vi "UI.Connection.State.Get.vi"(6 "Menu Ref":refnum<k9>, 7 "Name Ref":refnum<vi>, 8 "error in (no error)":errorcluster, 9 "Addon Path in":string, 10 "NIVS.System Definition Root in":refnum<k24>, 11 "NIVS.Workspace Ref in":T1) -> (0 "error out":errorcluster, 1 "Addon Connected?":bool, 2 "NIVS.System Definition Root out":refnum<k24>, 3 "NIVS.Workspace Ref out":T1)   [LabVIEW 2019, in "J1939 Workspace Shared.lvlib"]
uses:
  J1939 Workspace Shared.lvlib
  <vilib>/NI VeriStand/Execution/Workspace/WorkspaceAPI.ctl
  NationalInstruments.VeriStand.ClientAPI
  NationalInstruments.VeriStand.SystemStorage
  NationalInstruments.VeriStand.SystemDefinitionAPI
  <vilib>/NI VeriStand/Execution/Workspace/NI_VS Workspace ExecutionAPI.lvlib
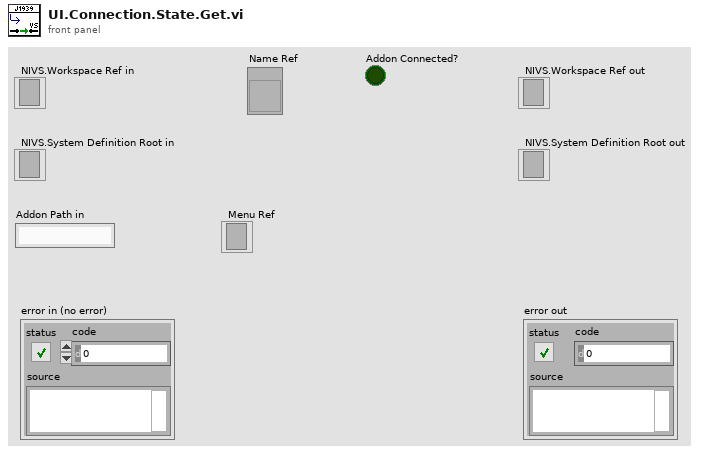
[diagram p1: front panel]
types:
  T1 = typedef "NI_VS Workspace ExecutionAPI.lvlib/WorkspaceAPI.ctl" = refnum<k24>
  T2 = typedef "NI_VS Workspace ExecutionAPI.lvlib/SystemState.ctl" = u8
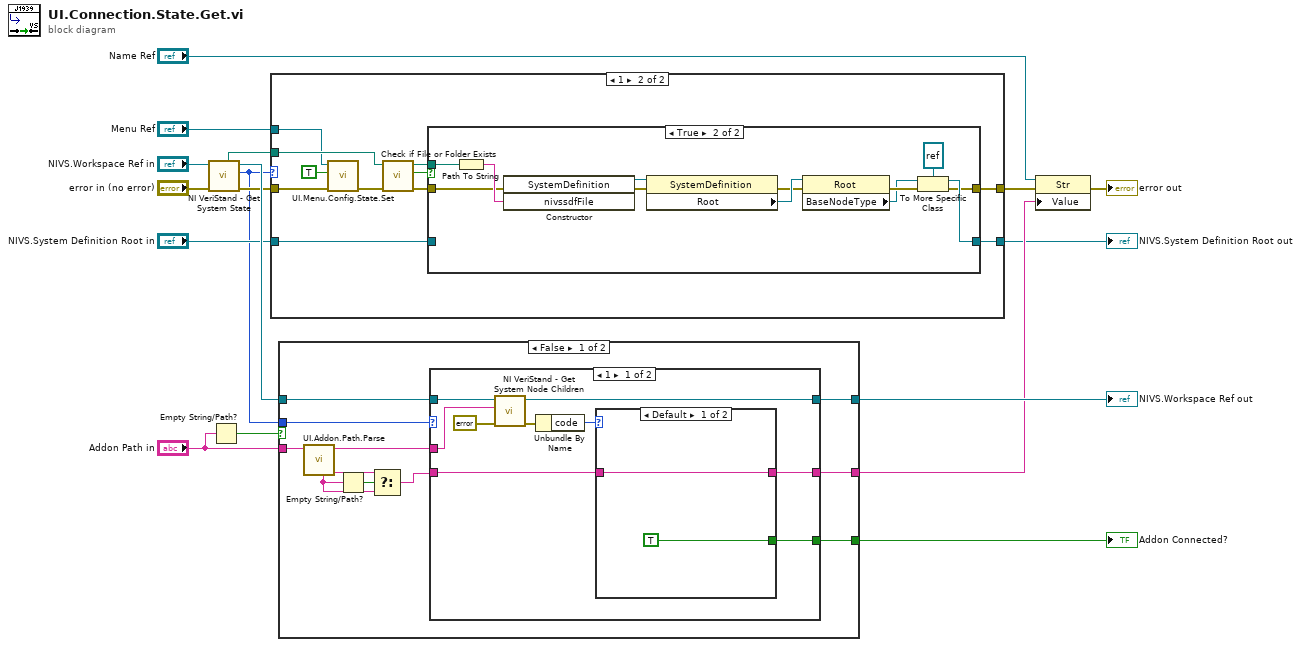
[diagram p0: block diagram]
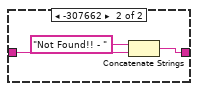
[diagram p2: hidden frame]
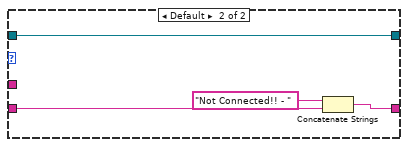
[diagram p3: hidden frame]
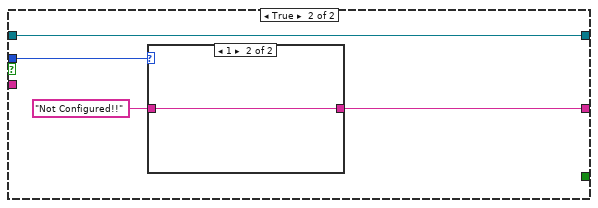
[diagram p4: hidden frame]
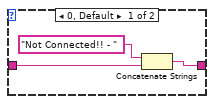
[diagram p5: hidden frame]
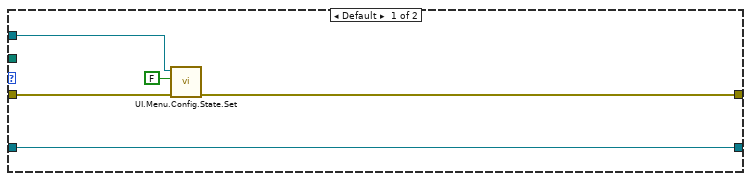
[diagram p6: hidden frame]
diagram:
  n1 = call <vilib>:"NI VeriStand - Get System State.vi"("error in (no error)"="error in (no error)", "WorkspaceManager in"="NIVS.Workspace Ref in") -> ("error out"=w5:errorcluster, "System State"=w2:T2, "WorkspaceManager  out"=w8:T1, "System Definition File"=w4:path)  [unwired: 5 in, 1 out]
  n2 = Empty String/Path?(string/path="Addon Path in") -> (empty?=w14:bool)
  n3 = case shown="1" w2 {
    tunnel: [w22 w33] -> w7
    tunnel: [w20 w32] -> w3
    tunnel: "NIVS.System Definition Root in" -> [w22 w29]
    tunnel: w5 -> [w19 w24]
    tunnel: w4 -> [_ w28]
    tunnel: "Menu Ref" -> [w18 w23]
    frame Default {
      n4 = call "UI.Menu.Config.State.Set.vi"("error in (no error)"=w19, "Enabled"=FALSE, "menu reference"=w18) -> ("error out"=w20:errorcluster)  [unwired: 8 in]
    }
    frame 1 {
      n5 = call "UI.Menu.Config.State.Set.vi"("error in (no error)"=w24, "Enabled"=TRUE, "menu reference"=w23) -> ("error out"=w25:errorcluster)  [unwired: 8 in]
      n6 = call <vilib>:"Check if File or Folder Exists.vi"("error in (no error)"=w25, "path"=w28) -> ("error out"=w31:errorcluster, "file or folder exists?"=w30:bool, "dup path"=w27:path)  [unwired: 7 in]
      n7 = case shown="True" w30 {
        tunnel: [w34 w37] -> w33
        tunnel: [w35 w36] -> w32
        tunnel: w31 -> [w35 w44]
        tunnel: w27 -> [_ w43]
        tunnel: w29 -> [w34 _]
        frame False {
        }
        frame True {
          n8 = Path To String(path=w43) -> (string=w46:string)
          n9 = constructor class="SystemDefinition"(error in=w44, "nivssdfFile"=w46) -> (reference out=w47:refnum<k24>, error out=w45:errorcluster)  [unwired: 2 in, 2 out]
          n10 = property class="SystemDefinition"(reference=w47, error in=w45) -> (error out=w38:errorcluster, "Root"=w39:refnum<k24>)  [unwired: 1 out]
          n11 = property class="Root"(reference=w39, error in=w38) -> (error out=w42:errorcluster, "BaseNodeType"=w41:refnum<k24>)  [unwired: 1 out]
          n12 = To More Specific Class(target class=refnum<k24> refnum, reference=w41, error in=w42) -> (specific class reference=w37:refnum<k24>, error out=w36:errorcluster)
        }
      }
    }
  }
  "NIVS.System Definition Root out" <- w7
  n13 = case shown="False" w14 {
    tunnel: [w58 w77] -> w12
    tunnel: [w57 w80] -> w17
    tunnel: "Addon Path in" -> [w53 _]
    tunnel: [w56 _] -> w13
    tunnel: w2 -> [w54 w79]
    tunnel: w8 -> [w55 w80]
    frame False {
      n14 = call "UI.Addon.Path.Parse.vi"("Cached Addon Path"=w53) -> ("Addon Name"=w49:string, "Addon Path"=w52:string, "Remaining Path"=w50:string)  [unwired: 6 in, 2 out]
      n15 = Empty String/Path?(string/path=w50) -> (empty?=w51:bool)
      n16 = Select(t=w49, s=w51, f=w50) -> (s? t:f=w48:string)
      n17 = case shown="1" w54 {
        tunnel: [w67 w76] -> w58
        tunnel: w48 -> [w66 w74]
        tunnel: [w63 w75] -> w57
        tunnel: [w62 _] -> w56
        tunnel: w55 -> [w61 w75]
        tunnel: w52 -> [w59 _]
        frame 1 {
          n18 = call <vilib>:"NI VeriStand - Get System Node Children.vi"("error in (no error)"=errorcluster {"status"=FALSE, "code"=0, "source"=""}, "Node"=w59, "WorkspaceManager in"=w61) -> ("error out"=w65:errorcluster, "WorkspaceManager out"=w63:T1)  [unwired: 6 in, 1 out]
          n19 = Unbundle By Name(w65) -> ("code"=w64:i32)
          n20 = case shown="Default" w64 {
            tunnel: w66 -> [w69 w71]
            tunnel: [w69 w72] -> w67
            tunnel: [TRUE _] -> w62
            frame Default {
            }
            frame -307662 {
              n21 = Concatenate Strings("Not Found!! - " ("string"), w71) -> (w72:string)
            }
          }
        }
        frame Default {
          n22 = Concatenate Strings("Not Connected!! - " ("string"), w74) -> (w76:string)
        }
      }
    }
    frame True {
      n23 = case shown="1" w79 {
        tunnel: [w82 w84] -> w77
        tunnel: "Not Configured!!" ("CD Path in") -> [w83 w84]
        frame 0, Default {
          n24 = Concatenate Strings("Not Connected!! - " ("string"), w83) -> (w82:string)
        }
        frame 1 {
        }
      }
    }
  }
  "NIVS.Workspace Ref out" <- w17
  "Addon Connected?" <- w13
  n25 = property class="Str"(reference="Name Ref", error in=w3, "Value"=w12) -> (error out=→"error out":errorcluster)  [unwired: 1 out]
